vi "Processing Step.vi"(8 "error in (no error)":errorcluster, 11 "Route Handler in":refnum<class "Route Handler.lvclass">) -> (0 "error out":errorcluster, 2 "Step":T1[](array[typedef]), 3 "Route Handler out":refnum<class "Route Handler.lvclass">)   [LabVIEW 2020, in "HTTP Server.lvlib" / "Route Handler.lvclass"]
uses:
  Route Handler.lvclass
  Processing Step.ctl
  HTTP Server.lvlib
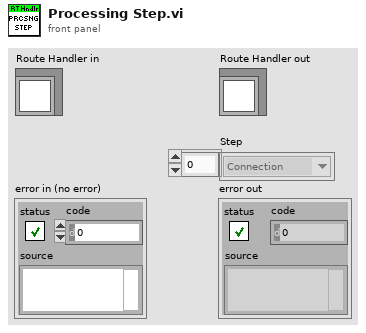
[diagram p1: front panel]
types:
  T1 = typedef "HTTP Server.lvlib/Processing Step.ctl" = enum16{"Connection", "Request", "Routing", "Controller Init", "Controller", "Response", "Complete", "Exception"}
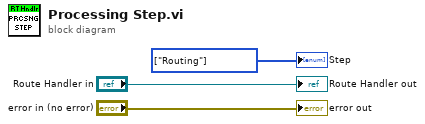
[diagram p0: block diagram]
diagram:
  w1 = T1[] [enum."Routing"] items=["Connection", "Request", "Routing", "Controller Init", "Controller", "Response", "Complete", "Exception"] ("Array")
  "error out" <- "error in (no error)"
  "Route Handler out" <- "Route Handler in"
  "Step" <- w1
